vi "print.vi"(6 "ShowType?":bool, 8 "error in (no error)":errorcluster, 11 "Expression":T1) -> (0 "error out":errorcluster, 3 "String":string)   [LabVIEW 2021]
uses:
  Expression.ctl
  ExpressionType.ctl
  ClosureData.ctl
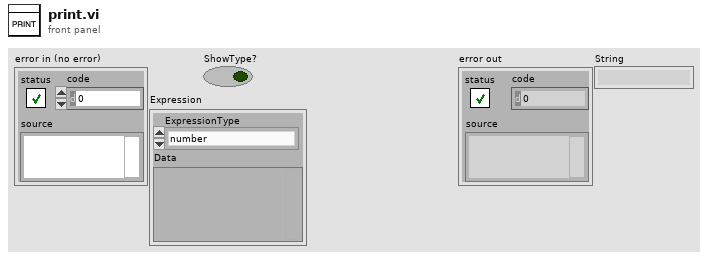
[diagram p1: front panel]
types:
  T1 = typedef "Expression.ctl" = cluster{"ExpressionType":T2, "Data":variant}
  T2 = typedef "ExpressionType.ctl" = enum16{"number", "string", "symbol", "primitive", "list", "closure", "nil", "error"}
  T3 = typedef "ClosureData.ctl" = cluster{"arguments":string[], "code":T1}
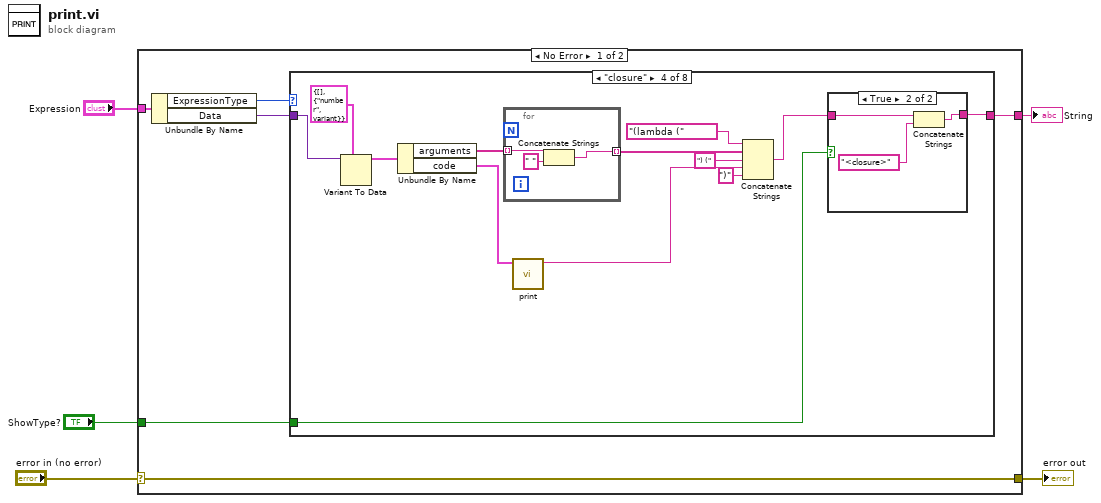
[diagram p0: block diagram]
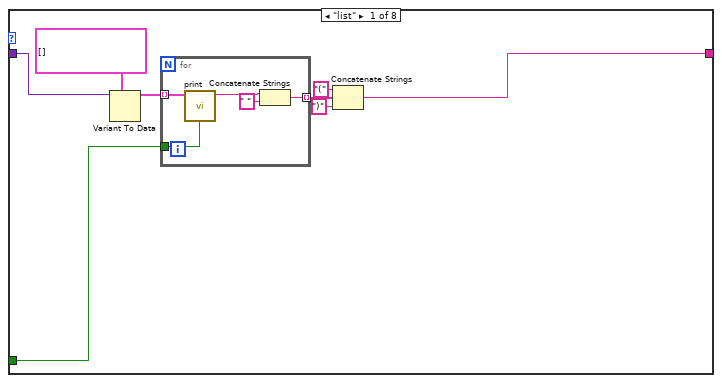
[diagram p2: hidden frame]
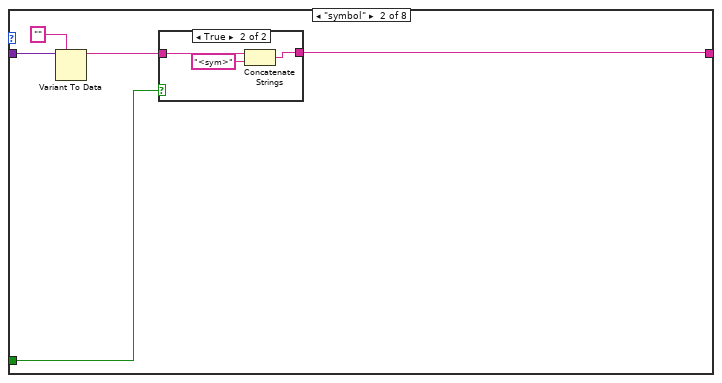
[diagram p3: hidden frame]
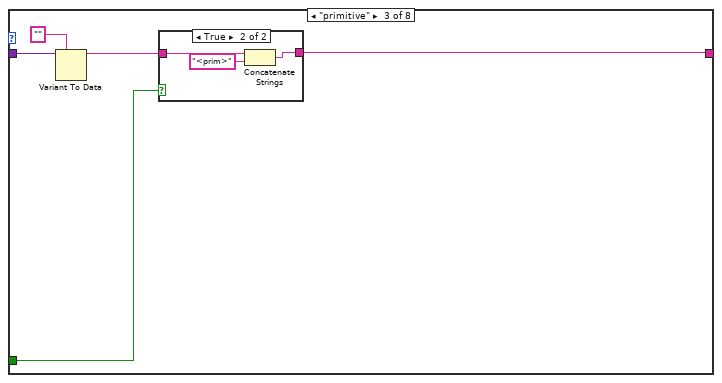
[diagram p5: hidden frame]
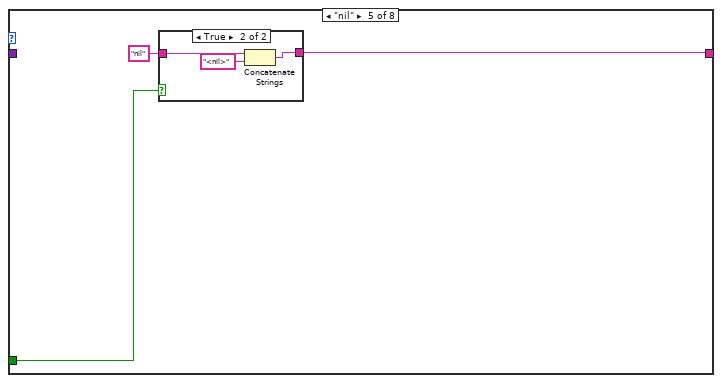
[diagram p8: hidden frame]
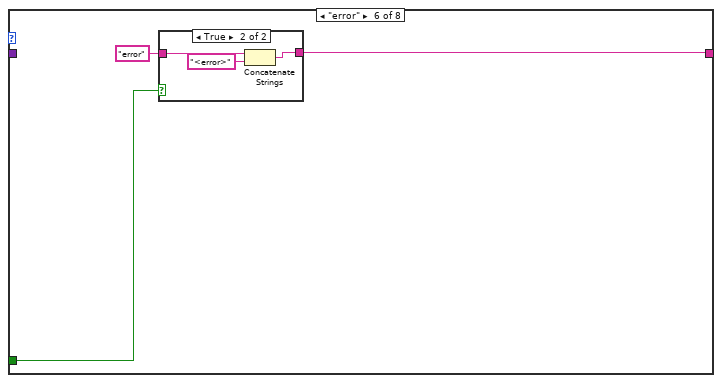
[diagram p10: hidden frame]
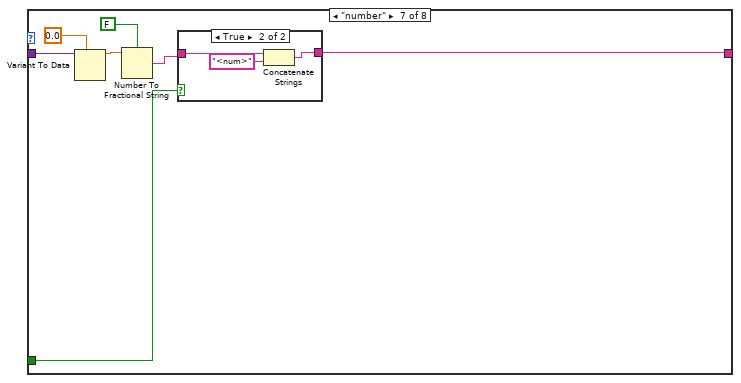
[diagram p12: hidden frame]
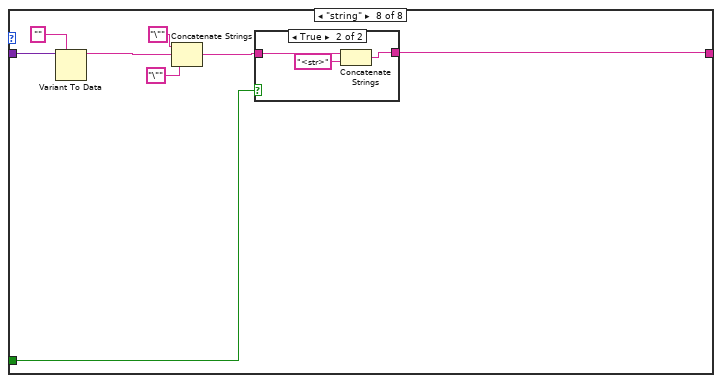
[diagram p14: hidden frame]
diagram:
  n1 = case shown="No Error" "error in (no error)" {
    selector: "error in (no error)" -> [w11 w100]
    tunnel: [w11 w100] -> w4
    tunnel: "Expression" -> [w10 _]
    tunnel: [w7 _] -> w3
    tunnel: "ShowType?" -> [w6 _]
    frame No Error {
      n2 = Unbundle By Name(w10) -> ("ExpressionType"=w9:T2, "Data"=w8:variant)
      n3 = case shown="\"closure\"" w9 {
        tunnel: w8 -> [w19 w29 w38 w55 _ _ w83 w95]
        tunnel: [w14 w26 w35 w54 w65 w72 w82 w92] -> w7
        tunnel: w6 -> [w13 w25 w34 w53 w64 w71 w81 w93]
        frame "list" {
          n4 = Variant To Data(type=T1[] [], Variant=w19) -> (data=w18:T1[])  [unwired: 1 in, 1 out]
          n5 = for {
            tunnel: w18 -> [w22] mode=indexing
            tunnel: [w23] -> w17 mode=indexing
            tunnel: w13 -> [w21]
            n6 = call "print.vi"("ShowType?"=w21, "Expression"=w22) -> ("String"=w20:string)  [unwired: 8 in, 1 out]
            n7 = Concatenate Strings(w20, " " ("string")) -> (w23:string)
          }
          n8 = Concatenate Strings("(" ("string"), w17, ")" ("string")) -> (w14:string)
        }
        frame "symbol" {
          n9 = Variant To Data(type="", Variant=w29) -> (data=w27:string)  [unwired: 1 in, 1 out]
          n10 = case shown="True" w25 {
            tunnel: [w30 w32] -> w26
            tunnel: w27 -> [w30 w33]
            frame False {
            }
            frame True {
              n11 = Concatenate Strings(w33, "<sym>" ("string")) -> (w32:string)
            }
          }
        }
        frame "primitive" {
          n12 = Variant To Data(type="", Variant=w38) -> (data=w36:string)  [unwired: 1 in, 1 out]
          n13 = case shown="True" w34 {
            tunnel: [w39 w41] -> w35
            tunnel: w36 -> [w39 w42]
            frame False {
            }
            frame True {
              n14 = Concatenate Strings(w42, "<prim>" ("string")) -> (w41:string)
            }
          }
        }
        frame "closure" {
          n15 = Variant To Data(type=T3 {"arguments"=[], "code"={"ExpressionType"=enum."number", "Data"=variant}} ("ClosureData"), Variant=w55) -> (data=w51:T3)  [unwired: 1 in, 1 out]
          n16 = Unbundle By Name(w51) -> ("arguments"=w49:string[], "code"=w50:T1)
          n17 = for {
            tunnel: w49 -> [w57] mode=indexing
            tunnel: [w56] -> w46 mode=indexing
            n18 = Concatenate Strings(w57, " " ("string")) -> (w56:string)
          }
          n19 = call "print.vi"("Expression"=w50) -> ("String"=w45:string)  [unwired: 9 in, 1 out]
          n20 = Concatenate Strings("(lambda (" ("string"), w46, ") (" ("string"), w45, ")" ("string")) -> (w43:string)
          n21 = case shown="True" w53 {
            tunnel: [w59 w62] -> w54
            tunnel: w43 -> [w59 w60]
            frame False {
            }
            frame True {
              n22 = Concatenate Strings(w60, "<closure>" ("string")) -> (w62:string)
            }
          }
        }
        frame "nil" {
          n23 = case shown="True" w64 {
            tunnel: [w66 w68] -> w65
            tunnel: "nil" -> [w66 w69]
            frame False {
            }
            frame True {
              n24 = Concatenate Strings(w69, "<nil>" ("string")) -> (w68:string)
            }
          }
        }
        frame "error" {
          n25 = case shown="True" w71 {
            tunnel: [w73 w75] -> w72
            tunnel: "error" -> [w73 w76]
            frame False {
            }
            frame True {
              n26 = Concatenate Strings(w76, "<error>" ("string")) -> (w75:string)
            }
          }
        }
        frame "number" {
          n27 = Variant To Data(type=0.0, Variant=w83) -> (data=w79:dbl)  [unwired: 1 in, 1 out]
          n28 = Number To Fractional String(use system decimal point (T)=FALSE, number=w79) -> (F-format string=w78:string)  [unwired: 2 in]
          n29 = case shown="True" w81 {
            tunnel: [w84 w86] -> w82
            tunnel: w78 -> [w84 w87]
            frame False {
            }
            frame True {
              n30 = Concatenate Strings(w87, "<num>" ("string")) -> (w86:string)
            }
          }
        }
        frame "string" {
          n31 = Variant To Data(type="", Variant=w95) -> (data=w89:string)  [unwired: 1 in, 1 out]
          n32 = Concatenate Strings("\"" ("string"), w89, "\"" ("string")) -> (w88:string)
          n33 = case shown="True" w93 {
            tunnel: [w96 w98] -> w92
            tunnel: w88 -> [w96 w99]
            frame False {
            }
            frame True {
              n34 = Concatenate Strings(w99, "<str>" ("string")) -> (w98:string)
            }
          }
        }
      }
    }
    frame Error {
      # "Wire the error cluster across even in the \"No Error\"\ncase so that warnings get propagated."
    }
  }
  "error out" <- w4
  "String" <- w3
